vi "VIs in memory.vi"() -> ()   [LabVIEW 2015]
panel:
  out "size(s)":i32
  out "Application:All VIs In Memory":string[](array[string])
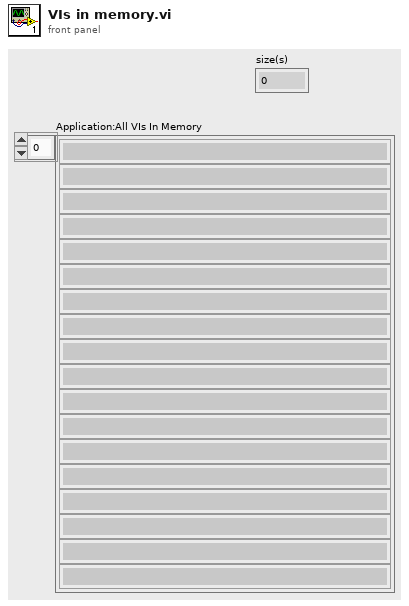
[diagram p1: front panel]
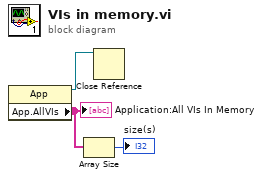
[diagram p0: block diagram]
diagram:
  n1 = property class="App"() -> (reference out=w3:refnum<vi>, "App.AllVIs"=w2:string[])  [unwired: 2 in, 1 out]
  "Application:All VIs In Memory" <- w2
  n2 = Array Size(array=w2) -> (size(s)=→"size(s)":i32)
  n3 = Close Reference(reference=w3) -> ()  [unwired: 1 in, 1 out]
